vi "Acquisition Message Loop.vi"(8 "error in (no error)":errorcluster, 9 "Data Queue":refnum<queue>, 10 "Data Notifier":refnum<notifier>, 11 "Message Queues":T1) -> (0 "error out":errorcluster)   [LabVIEW 2022 SP3, in "Acquisition.lvlib"]
doc: "Message loop for handling messages pertaining to the acquisition of data from the hardware."
uses:
  Acquisition.lvlib
  support/Message Queue/All Message Queues.ctl
  support/Message Queue/Message Cluster.ctl
  Network JSON.ctl
  Network Configuration.ctl
  Acquisition State.ctl
  support/Message Queue/Enqueue Message (Single).vi
  <vilib>/Utility/error.llb/Error Cluster From Error Code.vi
  <vilib>/ErrorRing/Error Ring.xnode
  support/Message Queue/Message Queue.lvlib
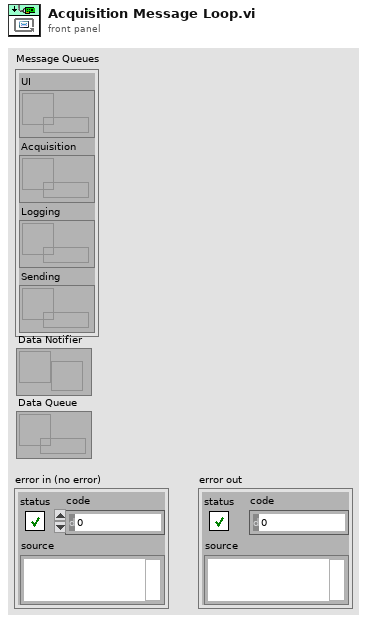
[diagram p1: front panel]
types:
  T1 = typedef "Message Queue.lvlib/All Message Queues.ctl" = cluster{"UI":refnum<queue>, "Acquisition":refnum<queue>, "Logging":refnum<queue>, "Sending":refnum<queue>}
  T2 = typedef "Acquisition.lvlib/Network Configuration.ctl" = cluster{"IP Address":string, "Port":dbl, "TCP Network Connection Refnum":refnum<k5>}
  T3 = typedef "Acquisition.lvlib/Acquisition State.ctl" = enum16{"Idle", "Acquiring"}
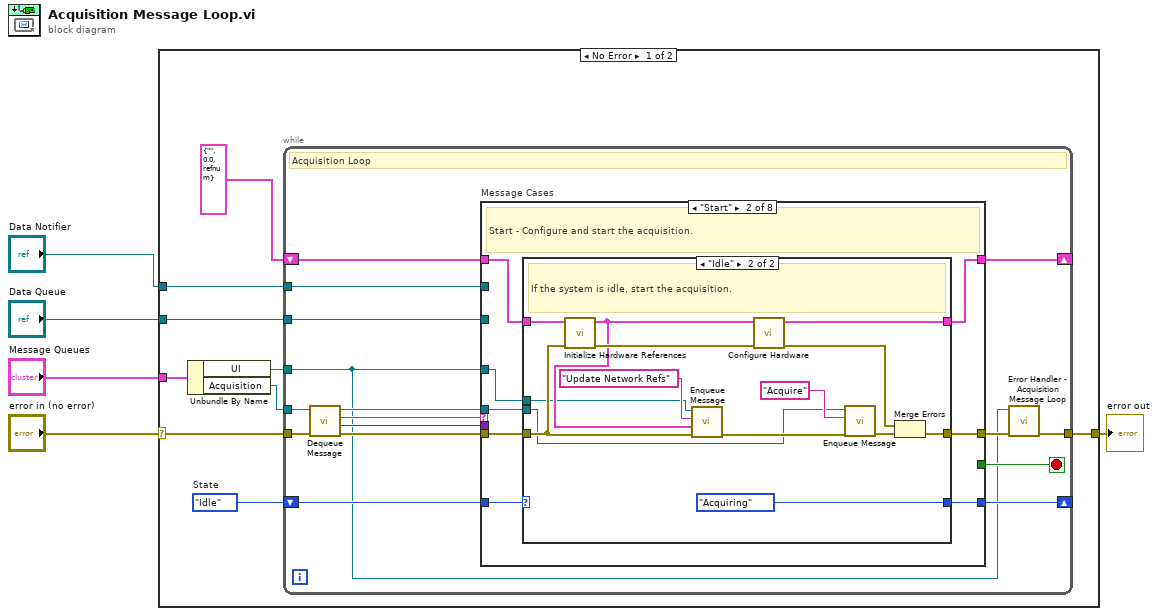
[diagram p0: block diagram]
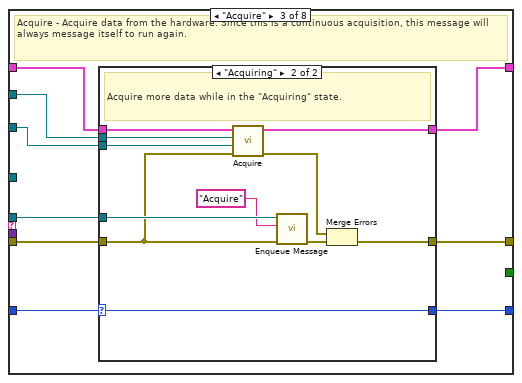
[diagram p4: hidden frame]
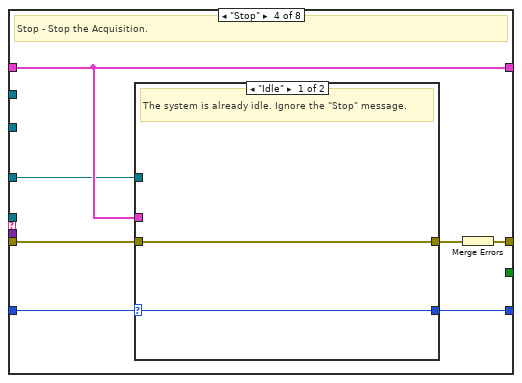
[diagram p6: hidden frame]
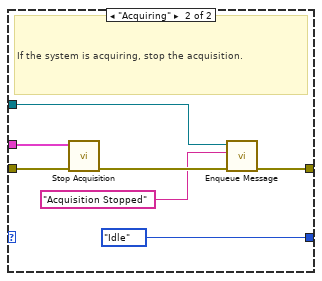
[diagram p7: hidden frame]
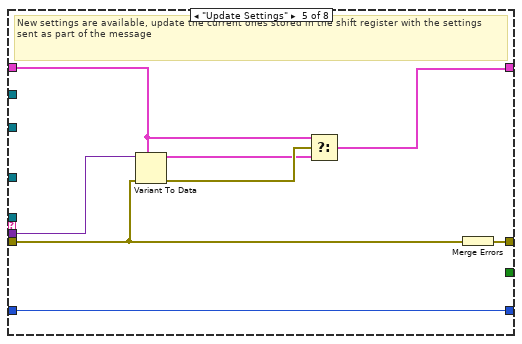
[diagram p8: hidden frame]
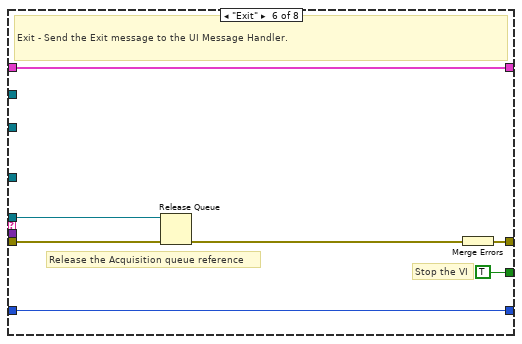
[diagram p9: hidden frame]
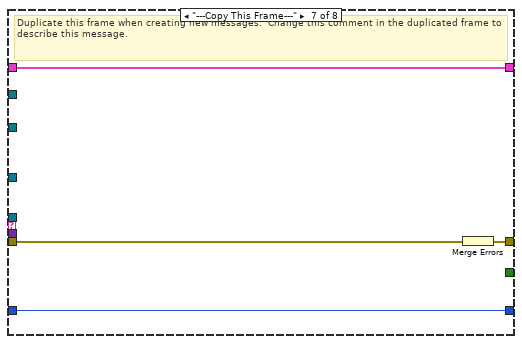
[diagram p10: hidden frame]
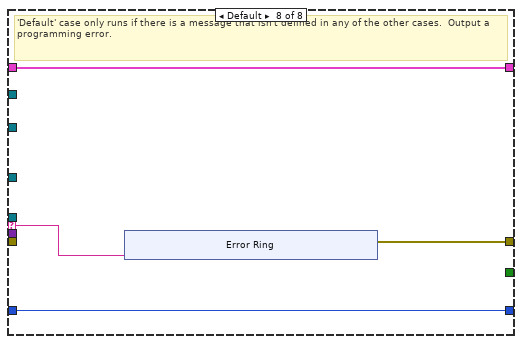
[diagram p11: hidden frame]
diagram:
  n1 = case shown="No Error" "error in (no error)" {
    selector: "error in (no error)" -> [w10 w128]
    tunnel: "Message Queues" -> [w14 _]
    tunnel: [w12 w128] -> w4
    tunnel: "Data Notifier" -> [w8 _]
    tunnel: "Data Queue" -> [w7 _]
    frame No Error {
      w6 = Acquisition_State."Idle"  # State
      n2 = Unbundle By Name(w14) -> ("UI"=w9:refnum<queue>, "Acquisition"=w13:refnum<queue>)
      n3 = while {
        tunnel: w13 -> [w23]
        shift-right: [w29] -> _
        shift-left: T2 {"IP Address"="", "Port"=0.0, "TCP Network Connection Refnum"=refnum} ("Data Cluster") -> [w30]
        tunnel: w9 -> [w15]
        tunnel: w8 -> [w22]
        tunnel: w7 -> [w21]
        shift-right: [w19] -> _
        shift-left: w6 -> [w20]
        tunnel: w10 -> [w27]
        tunnel: [w18] -> w12
        stop <- w28 stop-if-true
        # "Acquisition Loop"
        n4 = call "Dequeue Message.vi"("error in (no error)"=w27, "Message Queue"=w23) -> ("error out"=w26:errorcluster, "Message Data"=w24:variant, "Message"=w25:string, "dup Message Queue"=w16:refnum<queue>)  [unwired: 6 in]
        n5 = case "Message Cases" shown="\"Start\"" w25 {
          selector: w25 -> [_ _ _ _ _ _ _ w117]
          tunnel: w16 -> [_ w38 w66 _ _ w107 _ _]
          tunnel: w26 -> [w31 w39 w65 w87 w99 w109 w116 _]
          tunnel: [w31 w41 w67 w88 w105 w111 w114 w118] -> w17
          tunnel: w30 -> [w32 w40 w63 w85 w101 w110 w115 w120]
          tunnel: [w32 w37 w64 w85 w100 w110 w115 w120] -> w29
          tunnel: [_ _ _ _ _ TRUE _ _] -> w28
          tunnel: w24 -> [_ _ _ _ w104 _ _ _]
          tunnel: w15 -> [_ w34 _ w82 _ _ _ _]
          tunnel: w22 -> [_ _ w62 _ _ _ _ _]
          tunnel: w21 -> [_ _ w61 _ _ _ _ _]
          tunnel: w20 -> [w33 w35 w59 w84 w98 w106 w113 w119]
          tunnel: [w33 w36 w60 w83 w98 w106 w113 w119] -> w19
          frame "Initialize" {
            # "Initialize  - Initialize is currently a no-op.  The hardware initialization takes place in the 'Start' message."
          }
          frame "Start" {
            # "Start - Configure and start the acquisition."
            n6 = case shown="\"Idle\"" w35 {
              selector: w35 -> [w42 _]
              tunnel: [w43 w58] -> w41
              tunnel: w40 -> [w44 w57]
              tunnel: w39 -> [w43 w50]
              tunnel: w38 -> [_ w45]
              tunnel: [w44 w53] -> w37
              tunnel: [w42 Acquisition_State."Acquiring" ("Acquisition State")] -> w36
              tunnel: w34 -> [_ w46]
              frame "Acquiring" {
                # "The system is already acquiring. Ignore the \"Start\" message."
              }
              frame "Idle" {
                # "If the system is idle, start the acquisition."
                n7 = call "Initialize Hardware References.vi"("error in (no error)"=w50, "Hardware Resources in"=w57) -> ("error out"=w55:errorcluster, "Hardware Resources out"=w47:T2)  [unwired: 8 in]
                n8 = call-poly "Enqueue Message.vi"("error in (no error)"=w50, "Message Data"=w47, "Message"="Update Network Refs", "Message Queue"=w46) -> ("error out"=w49:errorcluster)  [unwired: 6 in, 1 out]
                n9 = call "Configure Hardware.vi"("error in (no error)"=w55, "Hardware Resources in"=w47) -> ("error out"=w54:errorcluster, "Hardware Resources out"=w53:T2)  [unwired: 8 in]
                n10 = call-poly "Enqueue Message.vi"("error in (no error)"=w49, "Message"="Acquire", "Message Queue"=w45) -> ("error out"=w56:errorcluster)  [unwired: 7 in, 1 out]
                n11 = Merge Errors(w54, w56) -> (w58:errorcluster)
              }
            }
          }
          frame "Acquire" {
            # "Acquire - Acquire data from the hardware. Since this is a continuous acquisition, this message will always message itself to run again."
            n12 = case shown="\"Acquiring\"" w59 {
              selector: w59 -> [w68 w72]
              tunnel: [w69 w81] -> w67
              tunnel: w66 -> [_ w79]
              tunnel: w65 -> [w69 w71]
              tunnel: [w70 w77] -> w64
              tunnel: w63 -> [w70 w76]
              tunnel: w62 -> [_ w74]
              tunnel: w61 -> [_ w73]
              tunnel: [w68 w72] -> w60
              frame "Idle" {
                # "Ignore \"Acquire\" messages when the acquisition is idle."
              }
              frame "Acquiring" {
                # "Acquire more data while in the \"Acquiring\" state."
                n13 = call "Acquire.vi"("error in (no error)"=w71, "Data Queue"=w73, "Data Notifier"=w74, "Hardware Resources in"=w76) -> ("error out"=w78:errorcluster, "Hardware Resources out"=w77:T2)  [unwired: 6 in]
                n14 = call-poly "Enqueue Message.vi"("error in (no error)"=w71, "Message"="Acquire", "Message Queue"=w79) -> ("error out"=w80:errorcluster)  [unwired: 7 in, 1 out]
                n15 = Merge Errors(w78, w80) -> (w81:errorcluster)
              }
            }
          }
          frame "Stop" {
            # "Stop - Stop the Acquisition."
            n16 = case shown="\"Idle\"" w84 {
              selector: w84 -> [w89 _]
              tunnel: w87 -> [w90 w97]
              tunnel: [w90 w93] -> w86
              tunnel: w85 -> [_ w95]
              tunnel: [w89 Acquisition_State."Idle" ("State")] -> w83
              tunnel: w82 -> [_ w92]
              frame "Idle" {
                # "The system is already idle. Ignore the \"Stop\" message."
              }
              frame "Acquiring" {
                # "If the system is acquiring, stop the acquisition."
                n17 = call "Stop Acquisition.vi"("error in (no error)"=w97, "Hardware Resources in"=w95) -> ("error out"=w96:errorcluster)  [unwired: 9 in]
                n18 = call-poly "Enqueue Message.vi"("error in (no error)"=w96, "Message"="Acquisition Stopped", "Message Queue"=w92) -> ("error out"=w93:errorcluster)  [unwired: 7 in, 1 out]
              }
            }
            n19 = Merge Errors(w86) -> (w88:errorcluster)
          }
          frame "Update Settings" {
            # "New settings are available, update the current ones stored in the shift register with the settings sent as part of the message"
            n20 = Variant To Data(error in=w99, type=w101, Variant=w104) -> (data=w102:T2, error out=w103:errorcluster)
            n21 = Select(t=w101, s=w103, f=w102) -> (s? t:f=w100:T2)
            n22 = Merge Errors(w99) -> (w105:errorcluster)
          }
          frame "Exit" {
            # "Release the Acquisition queue reference"
            # "Stop the VI"
            # "Exit - Send the Exit message to the UI Message Handler."
            n23 = Release Queue(queue=w107, error in (no error)=w109) -> (error out=w108:errorcluster)  [unwired: 1 in, 2 out]
            n24 = Merge Errors(w108) -> (w111:errorcluster)
          }
          frame "---Copy This Frame---" {
            # "Duplicate this frame when creating new messages.  Change this comment in the duplicated frame to describe this message."
            n25 = Merge Errors(w116) -> (w114:errorcluster)
          }
          frame Default {
            # "'Default' case only runs if there is a message that isn't defined in any of the other cases.  Output a programming error."
            n26 = xnode "Error Ring"("parameter 0"=w117) -> ("error out"=w118:errorcluster)
          }
        }
        n27 = call "Error Handler - Acquisition Message Loop.vi"("error in (no error)"=w17, "Message Queue"=w15) -> ("dup error in"=w18:errorcluster)  [unwired: 8 in, 1 out]
      }
    }
    frame Error {
    }
  }
  "error out" <- w4
